vi "T_kulso.vi"(9 "Parameterek":T1={"rholevego"=0.0, "Vlevego"=0.0, "Mlevego"=0.0, "clevego"=0.0, "rho PCM"=1100.0, "rho kulso"=28.3, "Dkulso"=0.1, "nkulso"=10, "dkulso"=0.0, "vkulso"=0.0, "rho kozepso"=28.3, "Dkozepso"=0.06, "nkozepso"=6, "dkozepso"=0.0, "vkozepso"=0.0, "mkozepso"=0.0, "mkulso"=0.0, "rho belso"=28.3, "Dbelso"=0.1, "nbelso"=10, "dbelso"=0.0, "vbelso"=0.0, "mbelso"=0.0, "Xpcm_kulso"=0.3, "Xpcm_belso"=0.3, "mpcm_kulso"=0.0, "mpcm_belso"=0.0, "mkulso_pcm"=0.0, "mbelso_pcm"=0.0, "ckulso"=1.13, "ckozepso"=1.13, "cbelso"=1.13, "cpcm_szilard"=1.9, "cpcm_foly"=1.5, "ckulso_Topalatt"=0.0, "cbelso_Topalatt"=0.0, "ckulso_Topfelett"=0.0, "cbelso_Topfelett"=0.0, "hpcm_olv"=140.0, "ckulso_eff_Tolv"=0.0, "cbelso_eff_Tolv"=0.0, "Qkulso_op_also"=0.0, "Qkulso_op_felso"=0.0, "Qbelso_op_also"=0.0, "Qbelso_op_felso"=0.0, "lambda_kulso"=5e-05, "lambda_kozepso"=5e-05, "lambda_belso"=5e-05, "lambda_pcm"=0.00018, "VXpcm_kulso"=0.0, "VXpcm_belso"=0.0, "lambda_kulsoPCM"=0.0, "lambda_belsoPCM"=0.0, "Alfa_kulso"=0.015, "Alfa_belso"=0.006, "Alfa_kont"=0.03, "Top_also"=24.0, "Top_felso"=28.0, "cpcm_olvnelkul"=0.0, "Tbelsolevego_0"=22.0}, 10 "Q kulso vektor":dbl[](array[numeric])) -> (2 "T kulso vektor":dbl[](array[numeric]))   [LabVIEW 2013]
uses:
  Parameterek.ctl
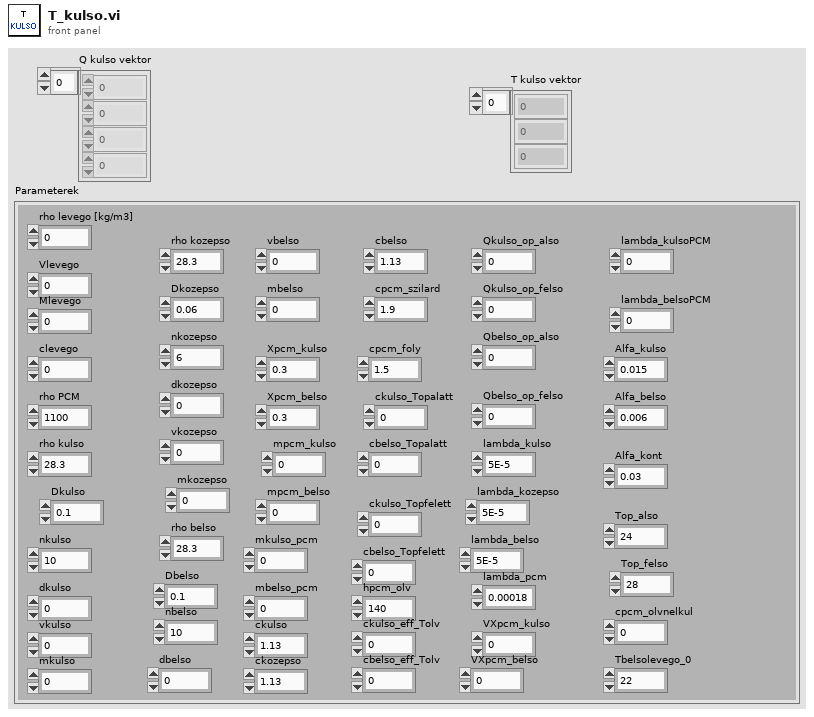
[diagram p1: front panel]
types:
  T1 = typedef "Parameterek.ctl" = cluster{"rholevego":dbl, "Vlevego":dbl, "Mlevego":dbl, "clevego":dbl, "rho PCM":dbl, "rho kulso":dbl, "Dkulso":dbl, "nkulso":i32, "dkulso":dbl, "vkulso":dbl, "rho kozepso":dbl, "Dkozepso":dbl, "nkozepso":i32, "dkozepso":dbl, "vkozepso":dbl, "mkozepso":dbl, "mkulso":dbl, "rho belso":dbl, "Dbelso":dbl, "nbelso":i32, "dbelso":dbl, "vbelso":dbl, "mbelso":dbl, "Xpcm_kulso":dbl, "Xpcm_belso":dbl, "mpcm_kulso":dbl, "mpcm_belso":dbl, "mkulso_pcm":dbl, "mbelso_pcm":dbl, "ckulso":dbl, "ckozepso":dbl, "cbelso":dbl, "cpcm_szilard":dbl, "cpcm_foly":dbl, "ckulso_Topalatt":dbl, "cbelso_Topalatt":dbl, "ckulso_Topfelett":dbl, "cbelso_Topfelett":dbl, "hpcm_olv":dbl, "ckulso_eff_Tolv":dbl, "cbelso_eff_Tolv":dbl, "Qkulso_op_also":dbl, "Qkulso_op_felso":dbl, "Qbelso_op_also":dbl, "Qbelso_op_felso":dbl, "lambda_kulso":dbl, "lambda_kozepso":dbl, "lambda_belso":dbl, "lambda_pcm":dbl, "VXpcm_kulso":dbl, "VXpcm_belso":dbl, "lambda_kulsoPCM":dbl, "lambda_belsoPCM":dbl, "Alfa_kulso":dbl, "Alfa_belso":dbl, "Alfa_kont":dbl, "Top_also":dbl, "Top_felso":dbl, "cpcm_olvnelkul":dbl, "Tbelsolevego_0":dbl}
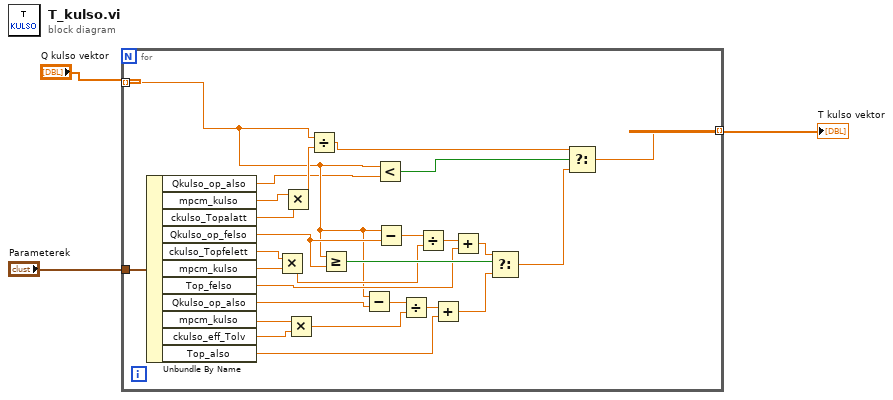
[diagram p0: block diagram]
diagram:
  n1 = for {
    tunnel: "Q kulso vektor" -> [w6] mode=indexing
    tunnel: [w28] -> w3 mode=indexing
    tunnel: "Parameterek" -> [w30]
    n2 = Unbundle By Name(w30) -> ("Qkulso_op_also"=w5:dbl, "mpcm_kulso"=w27:dbl, "ckulso_Topalatt"=w26:dbl, "Qkulso_op_felso"=w22:dbl, "ckulso_Topfelett"=w20:dbl, "mpcm_kulso"=w19:dbl, "Top_felso"=w15:dbl, "Qkulso_op_also"=w14:dbl, "mpcm_kulso"=w13:dbl, "ckulso_eff_Tolv"=w12:dbl, "Top_also"=w8:dbl)
    n3 = Multiply(x=w20, y=w19) -> (x*y=w18:dbl)
    n4 = Multiply(x=w27, y=w26) -> (x*y=w25:dbl)
    n5 = Multiply(x=w13, y=w12) -> (x*y=w10:dbl)
    n6 = Divide(x=w6, y=w25) -> (x/y=w29:dbl)
    n7 = Greater Or Equal?(x=w6, y=w22) -> (x >= y?=w24:bool)
    n8 = Subtract(x=w6, y=w14) -> (x-y=w11:dbl)
    n9 = Less?(x=w6, y=w5) -> (x < y?=w4:bool)
    n10 = Subtract(x=w6, y=w22) -> (x-y=w21:dbl)
    n11 = Divide(x=w11, y=w10) -> (x/y=w9:dbl)
    n12 = Divide(x=w21, y=w18) -> (x/y=w17:dbl)
    n13 = Add(x=w9, y=w8) -> (x+y=w7:dbl)
    n14 = Add(x=w17, y=w15) -> (x+y=w16:dbl)
    n15 = Select(t=w16, s=w24, f=w7) -> (s? t:f=w23:dbl)
    n16 = Select(t=w29, s=w4, f=w23) -> (s? t:f=w28:dbl)
  }
  "T kulso vektor" <- w3
